vi "read vendor name.vi"(8 "error in":errorcluster, 11 "Device in":refnum<class "Device.lvclass">) -> (0 "error out":errorcluster, 2 "vendor name":string, 3 "device out":refnum<class "Device.lvclass">)   [LabVIEW 2013, in "SMI.lvlib" / "Device.lvclass"]
uses:
  Device.lvclass
  Device.lvclass/Device.ctl
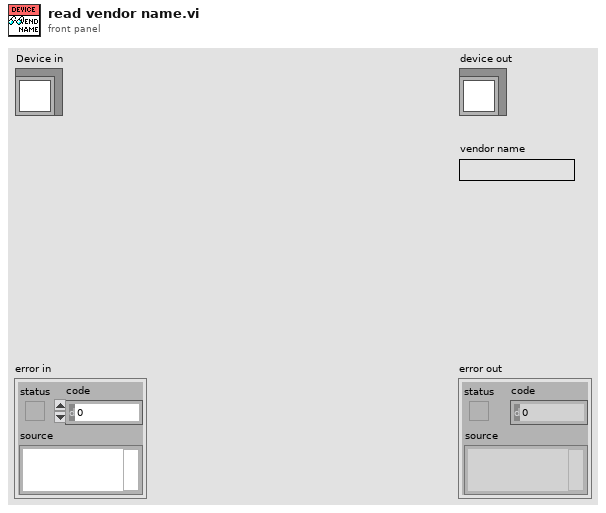
[diagram p1: front panel]
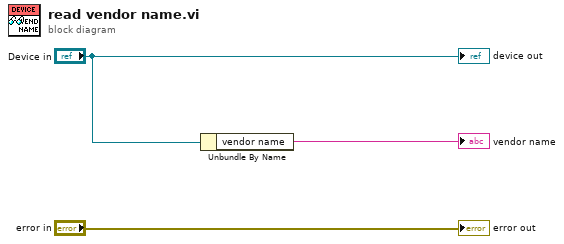
[diagram p0: block diagram]
diagram:
  n1 = Unbundle By Name("Device in") -> ("vendor name"=→"vendor name":string)
  "error out" <- "error in"
  "device out" <- "Device in"
